vi "WriteDataToReport.vi"(8 "error in":errorcluster, 11 "UI 1 Data":T1={"System Log"="", "[Array Of Threshold Refs]"=[], "[Array Of Boarder Refs]"=[], "APU Type"="", "APU Setup File"={"Sensor Info"=[], "Variables"=[], "CMM Table 106"=[], "CMM Table 106B "=[], "Accel Config"=[], "Report Sheet 1"=[], "Report Sheet 2"=[], "Report Sheet 3"=[]}, "ActiveValuetoRecordRow"=[], "ReportType"=[], "ReportValue"=[], "ActiveReportSheets"=[], "APUOn"=FALSE, "APUOnTime"=timestamp(0 s since 1904-01-01), "APUOffTime"=timestamp(0 s since 1904-01-01), "Recording"=FALSE, "Test Information"={"APU Part Number:"="555", "Model:"="5", "Serial Number:"="sad", "Customer:"="sad", "Work Order:"="asd", "Pre or Post SB"="Pre SB 49-7711", "Run Count"=0, "APU Selected"="<Select>"}, "APU RUN TIME"=timestamp(0 s since 1904-01-01)} {"APU RUN TIME" format="%<%H:%M:%S>T"; "Test Information"."Run Count" min=0 step=1; "APUOffTime" format="%<%x %.3X>T"; "APUOnTime" format="%<%x %.3X>T"}) -> (0 "error out":errorcluster)   [LabVIEW 2018, in "Testing UI 1.lvlib"]
uses:
  Testing UI 1.lvlib
  Private Controls/UI 1 Data.ctl
  Top Level/Shared Controls/APU Setup File.ctl
  File IO/Public Controls/ReportType.ctl
  Controller (Host)/Public Controls/Test Information.ctl
  Controller (Host)/Public VIs/PreorPostSB.ctl
  Controller (Host)/Public Controls/APU Select.ctl
  File IO/Public Controls/Write to Report.ctl
  File IO/Public Controls/Report Sheet Names.ctl
  File IO/File IO.lvlib
  Controller (Host)/Controller (Host).lvlib
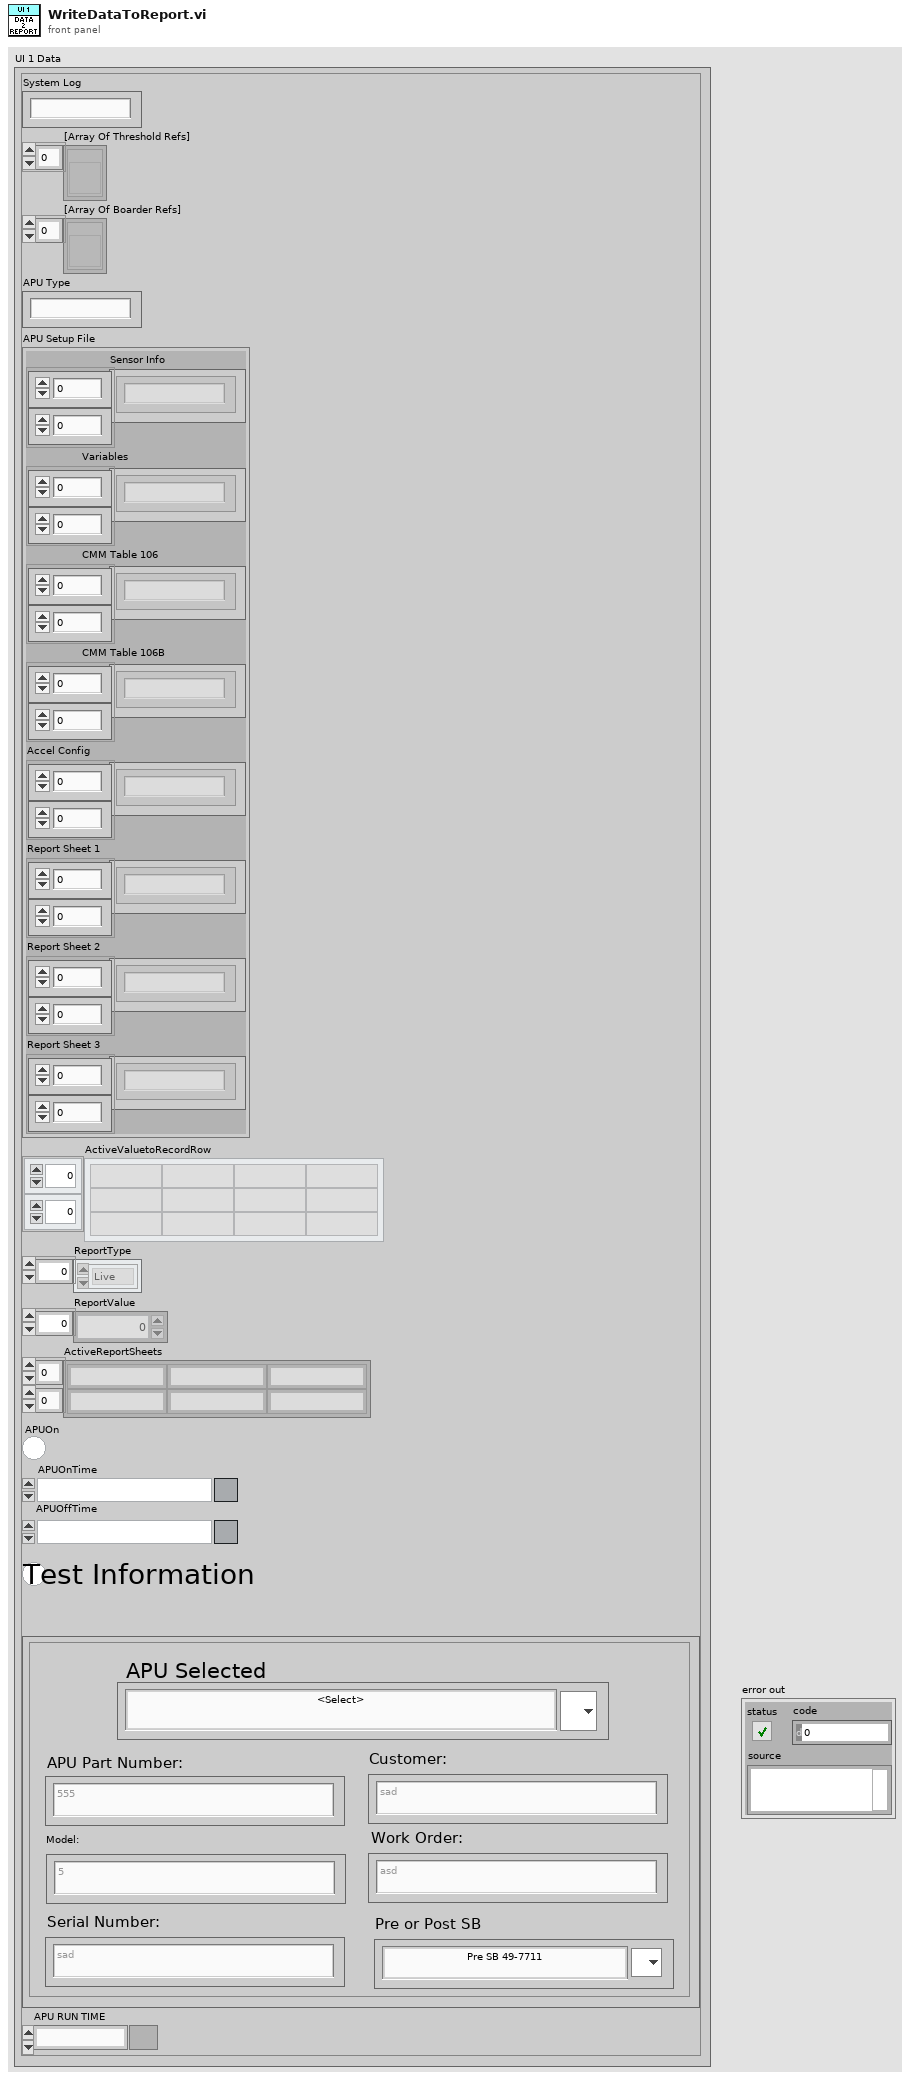
[diagram p1: front panel]
types:
  T1 = typedef "Testing UI 1.lvlib/UI 1 Data.ctl" = cluster{"System Log":string, "[Array Of Threshold Refs]":refnum<vi>[], "[Array Of Boarder Refs]":refnum<vi>[], "APU Type":string, "APU Setup File":T2, "ActiveValuetoRecordRow":string[][], "ReportType":T3[], "ReportValue":dbl[], "ActiveReportSheets":string[][], "APUOn":bool, "APUOnTime":timestamp, "APUOffTime":timestamp, "Recording":bool, "Test Information":T4, "APU RUN TIME":timestamp}
  T2 = typedef "APU Setup File.ctl" = cluster{"Sensor Info":string[][], "Variables":string[][], "CMM Table 106":string[][], "CMM Table 106B ":string[][], "Accel Config":string[][], "Report Sheet 1":string[][], "Report Sheet 2":string[][], "Report Sheet 3":string[][]}
  T3 = typedef "File IO.lvlib/ReportType.ctl" = enum16{"Live", "Min", "Max", "Deviation"}
  T4 = typedef "Controller (Host).lvlib/Test Information.ctl" = cluster{"APU Part Number:":string, "Model:":string, "Serial Number:":string, "Customer:":string, "Work Order:":string, "Pre or Post SB":T5, "Run Count":i32, "APU Selected":T6}
  T5 = typedef "Controller (Host).lvlib/PreorPostSB.ctl" = string
  T6 = typedef "Controller (Host).lvlib/APU Select.ctl" = string
  T7 = typedef "File IO.lvlib/Write to Report.ctl" = cluster{"Sheet Name":T8, "Cell #":string, "Data":string}
  T8 = typedef "File IO.lvlib/Report Sheet Names.ctl" = string
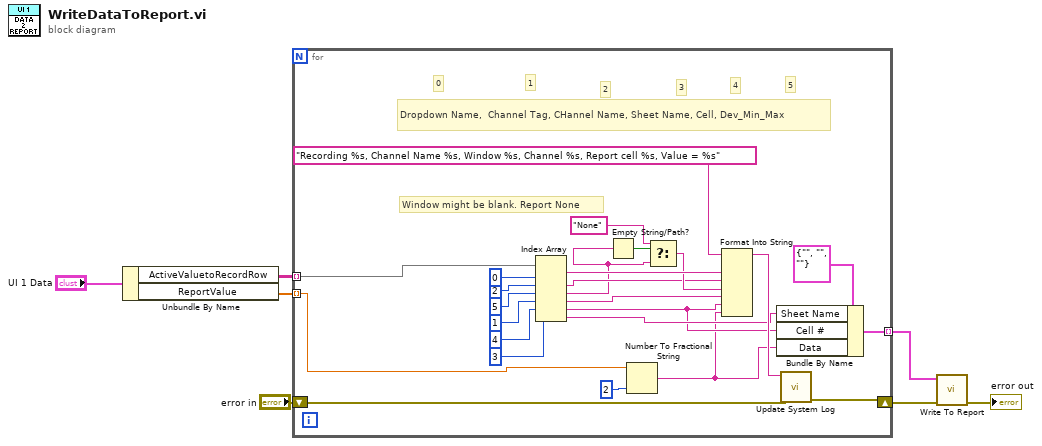
[diagram p0: block diagram]
diagram:
  n1 = Unbundle By Name("UI 1 Data") -> ("ActiveValuetoRecordRow"=w6:string[][], "ReportValue"=w7:dbl[])
  n2 = for {
    tunnel: w7 -> [w19] mode=indexing
    tunnel: w6 -> [w31] mode=indexing
    shift-right: [w23] -> w2
    shift-left: "error in" -> [w30]
    tunnel: [w29] -> w3 mode=indexing
    # "5"
    # "4"
    # "3"
    # "2"
    # "1"
    # "0"
    # "Dropdown Name,\t Channel Tag, CHannel Name,\tSheet Name, Cell, Dev_Min_Max"
    # "Window might be blank. Report None"
    n3 = Index Array(array=w31, index #1=0 ("index"), index #2=2 ("index"), index #3=5 ("index"), index #4=1 ("index"), index #5=4 ("index"), index #6=3 ("index")) -> (element #1=w28:string, element #2=w12:string, element #3=w11:string, element #4=w10:string, element #5=w9:string, element #6=w13:string)
    n4 = Empty String/Path?(string/path=w11) -> (empty?=w22:bool)
    n5 = Number To Fractional String(number=w19, precision (6)=i16 2) -> (F-format string=w8:string)  [unwired: 2 in]
    n6 = Select(t="None" ("element"), s=w22, f=w11) -> (s? t:f=w20:string)
    n7 = Format Into String(format string="Recording %s, Channel Name %s, Window %s, Channel %s, Report cell %s, Value = %s", w28, w12, w20, w10, w9, w8) -> (resulting string=w26:string)  [unwired: 2 in, 1 out]
    n8 = Bundle By Name(cluster=T7 {"Sheet Name"="", "Cell #"="", "Data"=""} ("Report Info"), "Sheet Name"=w13, "Cell #"=w9, "Data"=w8) -> (w29:T7)
    n9 = call "Update System Log.vi"("error in"=w30, "Message"=w26) -> ("error out"=w23:errorcluster)  [unwired: 9 in]
  }
  n10 = call "Write To Report.vi"("error in (no error)"=w2, "Report Info"=w3) -> ("error out"=→"error out":errorcluster)  [unwired: 9 in]
